vi "obtain_line_position_vector.vi"(8 "error in (no error)":errorcluster, 10 "line index (relative to frame)":i32, 11 "position channels":T2) -> (0 "error out":errorcluster, 3 "pixel positions":T1[](array[typedef]))   [LabVIEW 2010]
uses:
  common/classes/Image/Image/position_channels_cluster.ctl
  common/classes/Image/Image/Image.lvclass
  common/classes/ImageCollection/ImageCollection/pixel_position_cluster.ctl
  common/classes/ImageCollection/ImageCollection/ImageCollection.lvclass
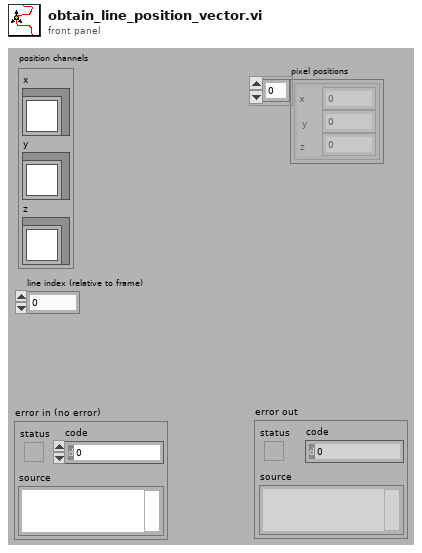
[diagram p1: front panel]
types:
  T1 = typedef "ImageCollection.lvclass/pixel_position_cluster.ctl" = cluster{"x":dbl, "y":dbl, "z ":dbl}
  T2 = typedef "Image.lvclass/position_channels_cluster.ctl" = cluster{"x":refnum<class "Image.lvclass">, "y":refnum<class "Image.lvclass">, "z":refnum<class "Image.lvclass">}
  T3 = typedef "IMAQ Image.ctl" = refnum<image>
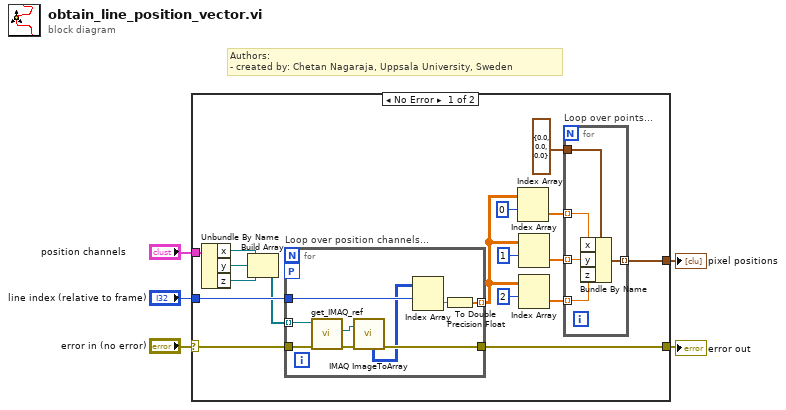
[diagram p0: block diagram]
diagram:
  # "Authors: \n- created by: Chetan Nagaraja, Uppsala University, Sweden"
  n1 = case shown="No Error" "error in (no error)" {
    selector: "error in (no error)" -> [w21 w37]
    tunnel: "position channels" -> [w22 _]
    tunnel: "line index (relative to frame)" -> [w20 _]
    tunnel: [w19 w37] -> w2
    tunnel: [w7 _] -> w1
    frame No Error {
      n2 = Unbundle By Name(w22) -> ("x"=w18:refnum<class "Image.lvclass">, "y"=w17:refnum<class "Image.lvclass">, "z"=w16:refnum<class "Image.lvclass">)
      n3 = Build Array(w18, w17, w16) -> (w15:refnum<class "Image.lvclass">[])
      n4 = for "Loop over position channels..." {
        tunnel: w21 -> [w35]
        tunnel: [w34] -> w13 mode=indexing
        tunnel: w20 -> [w33]
        tunnel: [w32] -> w19
        tunnel: w15 -> [w31] mode=indexing
        workers-P: _ -> [_]
        n5 = call-dynamic "get_IMAQ_ref.vi"("error in (no error)"=w35, "Image.lvclass in"=w31) -> ("error out"=w36:errorcluster, "Image"=w28:T3)  [unwired: 5 in, 3 out]
        n6 = call "IMAQ ImageToArray"("error in (no error)"=w36, "Image"=w28) -> ("Image Pixels (U16)"=w30:u16[][], "error out"=w32:errorcluster)  [unwired: 2 in, 3 out]
        n7 = Index Array(array=w30, index (row)=w33) -> (element=w29:u16[])  [unwired: 1 in]
        n8 = To Double Precision Float(number=w29) -> (double precision float=w34:dbl[])
      }
      n9 = Index Array(array=w13, index (row)=0) -> (element=w10:dbl[])  [unwired: 1 in]
      n10 = Index Array(array=w13, index (row)=1) -> (element=w9:dbl[])  [unwired: 1 in]
      n11 = Index Array(array=w13, index (row)=2) -> (element=w8:dbl[])  [unwired: 1 in]
      n12 = for "Loop over points..." {
        tunnel: w10 -> [w27] mode=indexing
        tunnel: w9 -> [w25] mode=indexing
        tunnel: w8 -> [w26] mode=indexing
        tunnel: T1 {"x"=0.0, "y"=0.0, "z "=0.0} ("position") -> [w24]
        tunnel: [w23] -> w7 mode=indexing
        n13 = Bundle By Name(cluster=w24, "x"=w27, "y"=w25, "z"=w26) -> (w23:T1)
      }
    }
    frame Error {
    }
  }
  "error out" <- w2
  "pixel positions" <- w1
